vi "Stop Response Complete.vi"(8 "error in (no error)":errorcluster, 11 "Monitor Controller in":refnum<class "Monitor Controller.lvclass">) -> (0 "error out":errorcluster, 3 "Monitor Controller out":refnum<class "Monitor Controller.lvclass">)   [LabVIEW 2018, in "Monitor Controller.lvclass"]
uses:
  Monitor Controller.lvclass
  C:/github/2018/LabActor/Worker/Worker.lvclass
  C:/github/2018/LabActor/Template Module/Template Module.lvclass
  C:/Program Files/National Instruments/LabVIEW 2018/vi.lib/ActorFramework/Actor/Actor.lvclass
  Worker/Worker.lvclass/Worker.ctl
  Template Module/Template Module.lvclass/Template Module.ctl
  <vilib>/ActorFramework/Message Enqueuer/Message Enqueuer.lvclass
  <vilib>/ActorFramework/Message Enqueuer/Message Enqueuer.lvclass/Message Enqueuer.ctl
  <vilib>/ActorFramework/Actor/Actor.lvclass/Actor.ctl
  Update Monitor State Msg/Update Monitor State Msg.lvclass/Update Monitor State Msg.ctl
  Template Module/Write Logger.vi
  Worker/Write Remote logger launched.vi
  Worker/Write Logger Enqueuer.vi
  Template Module/Read Logger.vi
  Worker/Read Use buffered logger.vi
  Worker/Read Remote logger launched.vi
  Worker/Read Logger Enqueuer.vi
  Template Module/Read State.vi
  <vilib>/ActorFramework/Message Enqueuer/Enqueue.vi
  <vilib>/ActorFramework/Stop Msg/Stop Msg.lvclass
  C:/Program Files/National Instruments/LabVIEW 2018/vi.lib/ActorFramework/Message/Message.lvclass
  Update Monitor State Msg/Update Monitor State Msg.lvclass
  <vilib>/ActorFramework/Message Priority Queue/Priority Enqueue.vi
  Loggers/Logger/Logger.lvclass
  Process Controller/Process Controller.lvclass
  <vilib>/ActorFramework/Actor/Actor.lvclass
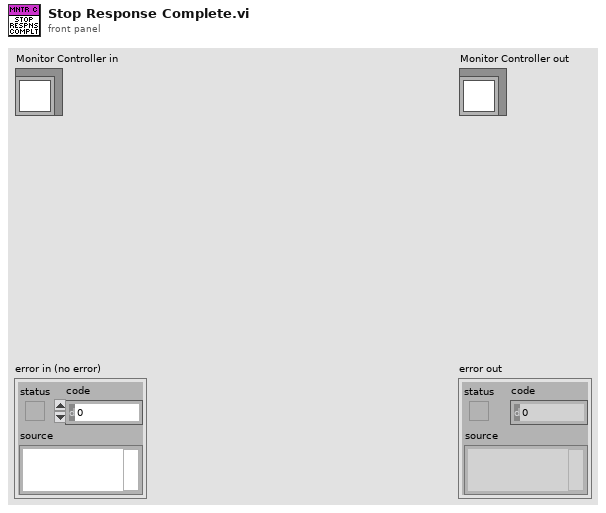
[diagram p1: front panel]
types:
  T1 = typedef "Worker State.ctl" = enum16{"Idle", "Starting", "Working", "Stopping"}
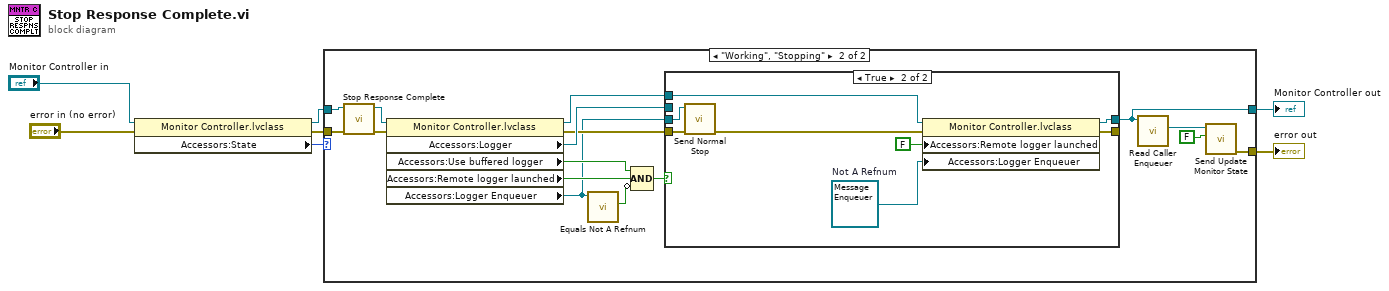
[diagram p0: block diagram]
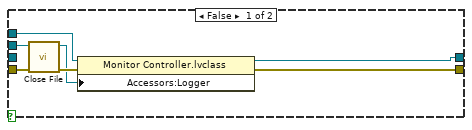
[diagram p3: hidden frame]
diagram:
  n1 = property class="Monitor Controller.lvclass"(reference="Monitor Controller in", error in="error in (no error)") -> (reference out=w6:refnum<class "Monitor Controller.lvclass">, error out=w7:errorcluster, "Accessors:State"=w5:T1)
  n2 = case shown="\"Working\", \"Stopping\"" w5 {
    tunnel: w7 -> [w8 w25]
    tunnel: w6 -> [w9 w24]
    tunnel: [w9 w10] -> w1
    tunnel: [w8 w23] -> w2
    frame "Idle", Default {
    }
    frame "Working", "Stopping" {
      n3 = call-parent "Stop Response Complete.vi"("error in (no error)"=w25, "Process Controller in"=w24) -> ("error out"=w11:errorcluster, "Process Controller out"=w12:refnum<class "Monitor Controller.lvclass">)  [unwired: 8 in]
      n4 = property class="Monitor Controller.lvclass"(reference=w12, error in=w11) -> (reference out=w20:refnum<class "Monitor Controller.lvclass">, error out=w18:errorcluster, "Accessors:Logger"=w19:refnum<class "Logger.lvclass">, "Accessors:Use buffered logger"=w16:bool, "Accessors:Remote logger launched"=w15:bool, "Accessors:Logger Enqueuer"=w13:refnum<class "Message Enqueuer.lvclass">)
      n5 = call <vilib>:"Equals Not A Refnum.vi"("Message Enqueuer"=w13) -> ("Not a refnum?"=w17:bool)  [unwired: 10 in]
      n6 = Compound Arithmetic op=AND(w16, w15, invert w17) -> (w14:bool)
      n7 = case shown="True" w14 {
        tunnel: [w32 w34] -> _
        tunnel: w20 -> [w31 w38]
        tunnel: [w30 w33] -> w10
        tunnel: w19 -> [w29 _]
        tunnel: w18 -> [w26 w39]
        tunnel: w13 -> [_ w40]
        frame False {
          n8 = call-dynamic "Close File.vi"("error in (no error)"=w26, "Logger in"=w29) -> ("error out"=w28:errorcluster, "Logger out"=w27:refnum<class "Logger.lvclass">)  [unwired: 6 in, 2 out]
          n9 = property class="Monitor Controller.lvclass"(reference=w31, error in=w28, "Accessors:Logger"=w27) -> (reference out=w30:refnum<class "Monitor Controller.lvclass">, error out=w32:errorcluster)
        }
        frame True {
          w35 = refnum<class "Message Enqueuer.lvclass"> refnum  # Not A Refnum
          n10 = call <vilib>:"Send Normal Stop.vi"("error in (no error)"=w39, "Message Enqueuer"=w40) -> ("error out"=w37:errorcluster)  [unwired: 9 in]
          n11 = property class="Monitor Controller.lvclass"(reference=w38, error in=w37, "Accessors:Remote logger launched"=FALSE ("Remote logger launched"), "Accessors:Logger Enqueuer"=w35) -> (reference out=w33:refnum<class "Monitor Controller.lvclass">, error out=w34:errorcluster)
        }
      }
      n12 = call <vilib>:"Read Caller Enqueuer.vi"("Actor"=w10) -> ("Caller Enqueuer"=w22:refnum<class "Message Enqueuer.lvclass">)  [unwired: 10 in]
      n13 = call "Send Update Monitor State.vi"("Monitor Running"=FALSE, "Message Enqueuer"=w22) -> ("error out"=w23:errorcluster)  [unwired: 8 in, 1 out]
    }
  }
  "error out" <- w2
  "Monitor Controller out" <- w1
